vi "equ_test.vi"() -> ()   [LabVIEW 2018]
uses:
  <vilib>/sound2/lvsound2.llb/Sampling Mode.ctl
  <vilib>/sound2/lvsound2.llb/Sound Data Format.ctl
  <vilib>/sound2/lvsound2.llb/Sound File Position.ctl
  <vilib>/sound2/lvsound2.llb/Sound File Read Open.vi
  <vilib>/sound2/lvsound2.llb/Sound File Read (DBL).vi
  <vilib>/sound2/lvsound2.llb/Sound Output Write (DBL).vi
panel:
  in  "Bypass":bool
  in  "Bajos":dbl(knob) scale=0.0..2.0
  in  "Medios":dbl(knob) scale=0.0..2.0
  in  "Agudos":dbl(knob) scale=0.0..2.0
  in  "Stop":bool
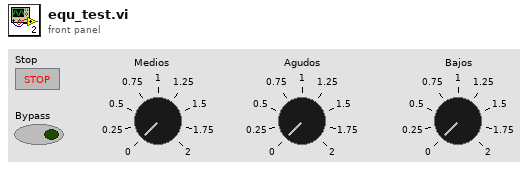
[diagram p1: front panel]
types:
  T1 = typedef "Sound Data Format.ctl" = cluster{"sample rate (S/s)":dbl, "number of channels":i32, "bits per sample":i32}
  T2 = typedef "Sampling Mode.ctl" = i32
  T3 = typedef "Sound Output Task ID.ctl" = u32
  T4 = typedef "Sound File Refnum.ctl" = refnum<file>
  T5 = typedef "Sound File Position.ctl" = u16
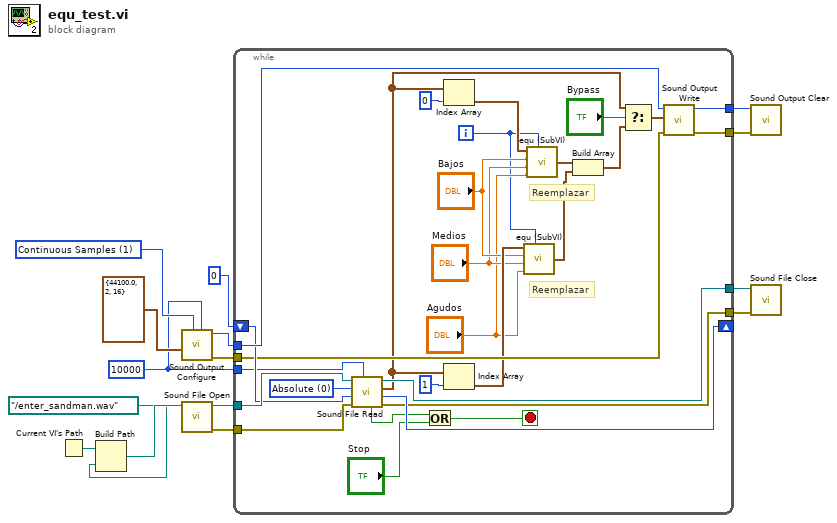
[diagram p0: block diagram]
diagram:
  w5 = 10000 ("number of samples/ch")
  w13 = T2 1 items=["Finite Samples", "Continuous Samples"] ("sample mode")
  n1 = Current VI's Path() -> (path=w3:path)
  n2 = Build Path(base path=w3, name or relative path=path "../enter_sandman.wav" ("path")) -> (appended path=w2:path)
  n3 = call <vilib>:"Sound Output Configure.vi"("number of samples/ch"=w5, "sample mode"=w13, "sound format"=T1 {"sample rate (S/s)"=44100.0, "number of channels"=2, "bits per sample"=16}) -> ("error out"=w9:errorcluster, "task ID"=w14:T3)  [unwired: 7 in]
  n4 = call-poly <vilib>:"Sound File Open.vi"("path"=w2) -> ("error out"=w8:errorcluster, "sound file refnum"=w15:T4)  [unwired: 9 in]
  n5 = while {
    tunnel: w15 -> [w44]
    tunnel: w14 -> [w43]
    shift-right: [w42] -> _
    shift-left: 0 ("offset") -> [w41]
    tunnel: [w39] -> w11
    tunnel: [w38] -> w10
    tunnel: w9 -> [w37]
    tunnel: w8 -> [w36]
    tunnel: [w35] -> w7
    tunnel: [w34] -> w6
    tunnel: w5 -> [w33]
    i -> [w16]
    stop <- w30 stop-if-true
    w40 = T5 0 items=["Absolute"=0, "Relative"=2] ("position mode")
    # "Reemplazar"
    # "Reemplazar"
    n6 = call-poly <vilib>:"Sound File Read.vi"("number of samples/ch (-1: all)"=w33, "error in (no error)"=w36, "position offset"=w41, "position mode"=w40, "sound file refnum"=w44) -> ("error out"=w34:errorcluster, "offset"=w42:i32, "data"=w27:waveform(dbl)[], "sound file refnum out"=w35:T4, "end of file?"=w32:bool)  [unwired: 2 in]
    n7 = Or(x=w32, y="Stop") -> (x .or. y?=w30:bool)
    n8 = Index Array(array=w27, index=0) -> (element=w21:waveform(dbl))
    n9 = Index Array(array=w27, index=1) -> (element=w23:waveform(dbl))
    n10 = call "equ (SubVI).vi"("Entrada"=w23, "Bajos"="Bajos", "Medios"="Medios", "Agudos"="Agudos", "Indice de Bloque"=w16) -> ("Salida"=w22:waveform(dbl))
    n11 = call "equ (SubVI).vi"("Entrada"=w21, "Bajos"="Bajos", "Medios"="Medios", "Agudos"="Agudos", "Indice de Bloque"=w16) -> ("Salida"=w17:waveform(dbl))
    n12 = Build Array(w17, w22) -> (w24:waveform(dbl)[])
    n13 = Select(t=w27, s="Bypass", f=w24) -> (s? t:f=w29:waveform(dbl)[])
    n14 = call-poly <vilib>:"Sound Output Write.vi"("error in (no error)"=w37, "data"=w29, "task ID"=w43) -> ("error out"=w38:errorcluster, "task ID out"=w39:T3)  [unwired: 7 in]
  }
  n15 = call <vilib>:"Sound Output Clear.vi"("error in (no error)"=w10, "task ID"=w11) -> ()  [unwired: 9 in, 1 out]
  n16 = call <vilib>:"Sound File Close.vi"("error in (no error)"=w6, "sound file refnum"=w7) -> ()  [unwired: 9 in, 1 out]
